vi "Digital Write 1 Channel.vi"(8 "error constant":errorcluster, 9 "Value":bool=TRUE, 10 "Channel":i32, 11 "NI-DAQ.lvclass":refnum<class "NI-DAQ.lvclass">) -> (0 "error IO":errorcluster, 3 "NI-DAQ.lvclass 2":refnum<class "NI-DAQ.lvclass">)   [LabVIEW 2016, in "NI-DAQ.lvclass"]
uses:
  NI-DAQ.lvclass
  NI-DAQ.lvclass/NI-DAQ.ctl
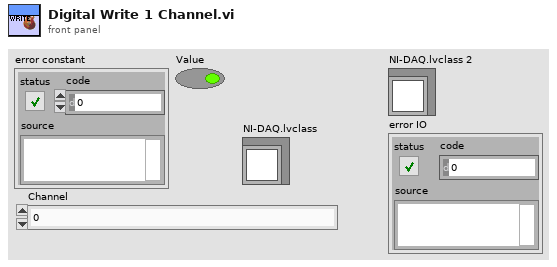
[diagram p1: front panel]
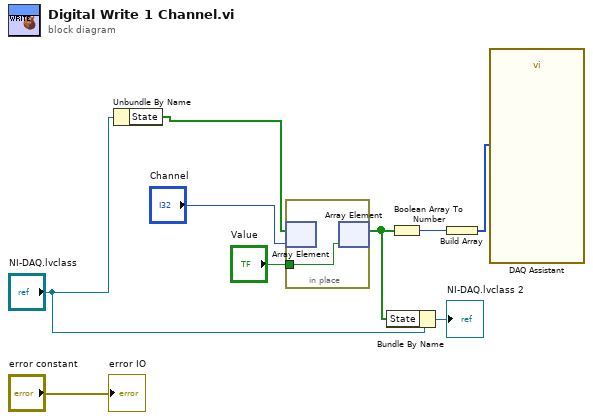
[diagram p0: block diagram]
diagram:
  n1 = Unbundle By Name("NI-DAQ.lvclass") -> ("State"=w1:bool[])
  n2 = in-place {
    in-place-border: "Value" -> [w10]
    n3 = in-place-array #1(w1, "Channel") -> ()  [unwired: 1 out]
    n4 = in-place-array #1(w10) -> (w2:bool[])  [unwired: 1 out]
  }
  n5 = Bundle By Name(cluster="NI-DAQ.lvclass", "State"=w2) -> (→"NI-DAQ.lvclass 2":refnum<class "NI-DAQ.lvclass">)
  n6 = Boolean Array To Number(Boolean array=w2) -> (number=w3:u32)
  n7 = Build Array(w3) -> (w5:u32[])
  n8 = call "DAQ Assistant"("data"=w5) -> ()  [unwired: 17 in, 2 out]
  "error IO" <- "error constant"
